vi "Host_GUI_Display_Image.vi"() -> ()   [LabVIEW 2017]
panel:
  in  "stop":bool
  out "Image":T1(plugin-control)
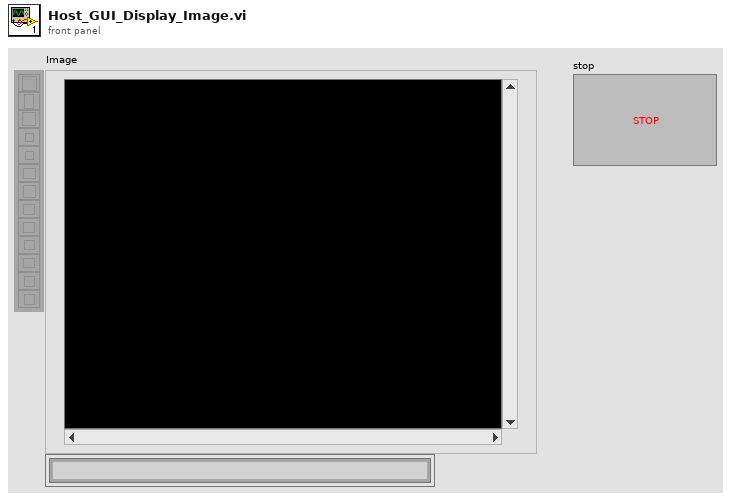
[diagram p1: front panel]
types:
  T1 = typedef "IMAQ Image.ctl" = refnum<image>
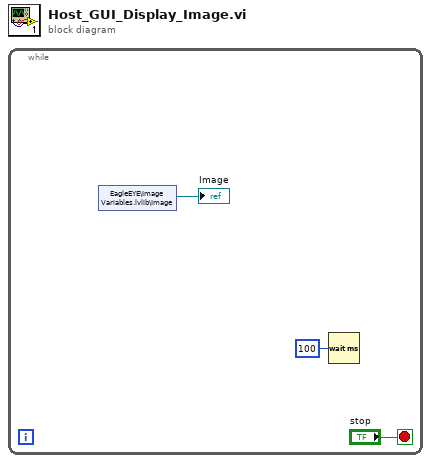
[diagram p0: block diagram]
diagram:
  n1 = while {
    stop <- "stop" stop-if-true
    n2 = shared-variable "EagleEYE\\Image Variables.lvlib\\Image"() -> (→"Image":refnum<image>)  [unwired: 1 in, 1 out]
    n3 = Wait (ms)(milliseconds to wait=u32 100) -> ()  [unwired: 1 out]
  }
